vi "Calculate Samples to Read for Each Iteration.vi"(10 "max samples to read at once":i32=1000000 format="%.0p", 11 "total samples to read":i32) -> (3 "samples to read":i32[](array[numeric]))   [LabVIEW 2021]
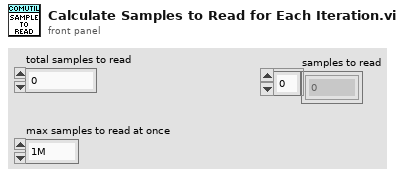
[diagram p1: front panel]
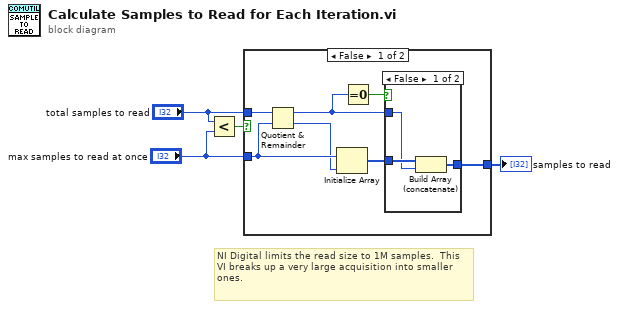
[diagram p0: block diagram]
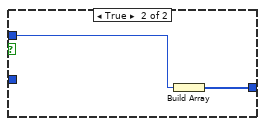
[diagram p3: hidden frame]
diagram:
  # "NI Digital limits the read size to 1M samples.  This VI breaks up a very large acquisition into smaller ones."
  n1 = Less?(x="total samples to read", y="max samples to read at once") -> (x < y?=w3:bool)
  n2 = case shown="False" w3 {
    tunnel: "total samples to read" -> [w11 w17]
    tunnel: "max samples to read at once" -> [w10 _]
    tunnel: [w8 w16] -> w1
    frame False {
      n3 = Quotient & Remainder(x=w11, y=w10) -> (x-y*floor(x/y)=w6:i32, floor(x/y)=w7:i32)
      n4 = Initialize Array(w10, w7) -> (w9:i32[])
      n5 = Equal To 0?(x=w6) -> (x = 0?=w5:bool)
      n6 = case shown="False" w5 {
        tunnel: w9 -> [w14 w15]
        tunnel: [w13 w15] -> w8
        tunnel: w6 -> [w12 _]
        frame False {
          n7 = Build Array (concatenate)(w14, w12) -> (w13:i32[])
        }
        frame True {
        }
      }
    }
    frame True {
      n8 = Build Array(w17) -> (w16:i32[])
    }
  }
  "samples to read" <- w1
